vi "CMI ckd2 Set Clock Source.vi"(8 "error in":errorcluster, 10 "clock source (auto)":T1, 11 "session":T2) -> (0 "error out":errorcluster, 3 "session out":T2)   [LabVIEW 2020, in "AWG.lvlib"]
doc: "Sets clock source of the clock divider."
uses:
  AWG.lvlib
  CMI ckd2 Session.ctl
  CMI ckd2 Source Mode.ctl
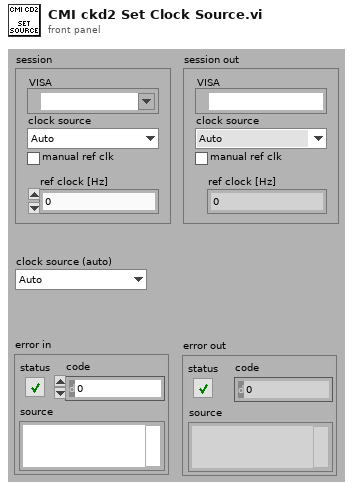
[diagram p1: front panel]
types:
  T1 = typedef "AWG.lvlib/CMI ckd2 Source Mode.ctl" = enum16{"Auto", "LF clock", "HF clock", "Internal"}
  T2 = typedef "AWG.lvlib/CMI ckd2 Session.ctl" = cluster{"VISA":refnum<visa-resource-name>, "clock source":T1, "manual ref clk":bool, "ref clock [Hz]":dbl}
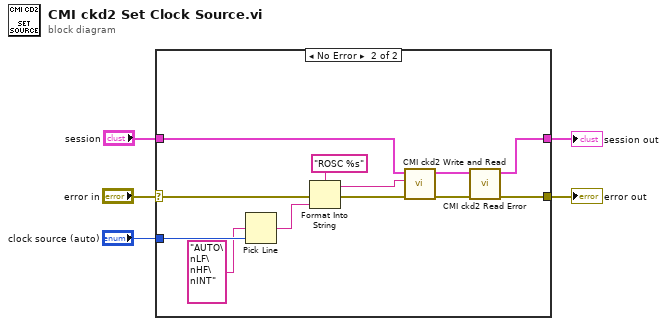
[diagram p0: block diagram]
diagram:
  n1 = case shown="No Error" "error in" {
    selector: "error in" -> [w6 w18]
    tunnel: [w7 w12] -> w3
    tunnel: [w6 w11] -> w5
    tunnel: "session" -> [w7 w19]
    tunnel: "clock source (auto)" -> [_ w10]
    frame Error {
    }
    frame No Error {
      n2 = Pick Line(multi-line string="AUTO\nLF\nHF\nINT", line index=w10) -> (output string=w9:string)  [unwired: 1 in]
      n3 = Format Into String(format string="ROSC %s", error in=w18, w9) -> (resulting string=w16:string, error out=w15:errorcluster)  [unwired: 1 in]
      n4 = call "CMI ckd2 Write and Read.vi"("error in"=w15, "command"=w16, "session"=w19) -> ("error out"=w14:errorcluster, "session out"=w13:T2)  [unwired: 6 in, 1 out]
      n5 = call "CMI ckd2 Read Error.vi"("error in"=w14, "session"=w13) -> ("error out"=w11:errorcluster, "session out"=w12:T2)  [unwired: 7 in, 1 out]
    }
  }
  "error out" <- w5
  "session out" <- w3
